vi "Make empty strings null.vi"(11 "JSON Input":string) -> (3 "<JSON>":string)   [LabVIEW 2020, in "JSONtext.lvlib"]
uses:
  <vilib>/JDP Science/JSONtext/JSONtext.lvlib
  <vilib>/JDP Science/JDP Science Common Utilities/JDP Utility.lvlib
panel:
  # "Make empty input count as null"
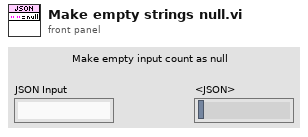
[diagram p1: front panel]
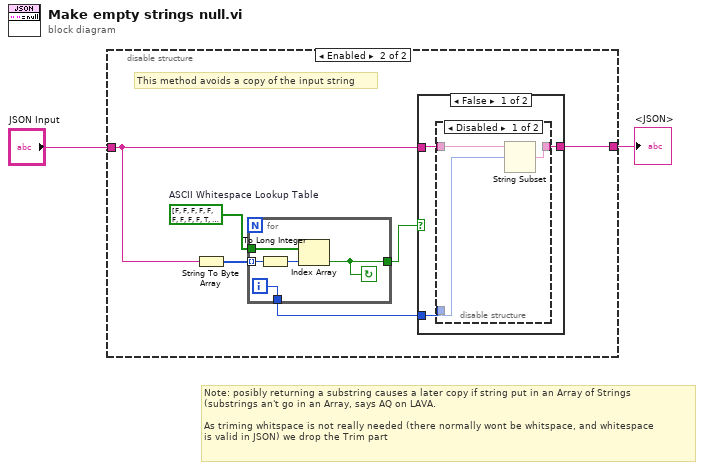
[diagram p0: block diagram]
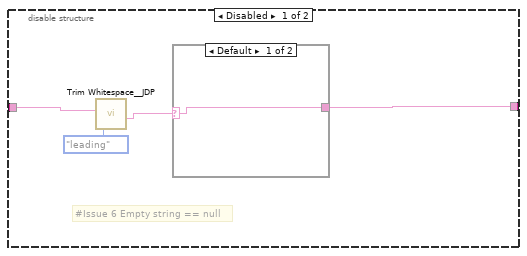
[diagram p2: hidden frame]
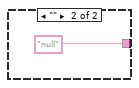
[diagram p3: hidden frame]
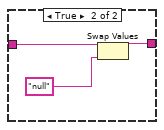
[diagram p5: hidden frame]
diagram:
  # "Note: posibly returning a substring causes a later copy if string put in an Array of Strings\n(substrings an't go in an Array, says AQ on LAVA.\n\nAs triming whitspace is not really needed (there normally wont be whitspace, and whitespace\nis valid in JSON) we drop the Trim part"
  n1 = disable-structure shown="Enabled" {
    disable-tunnel: "JSON Input" -> [w6 w12]
    disable-tunnel: [w4 w11] -> w1
    frame Disabled {
      # "#Issue 6 Empty string == null"
      n2 = call <vilib>:"Trim Whitespace__JDP.vi"("Remove (leading and trailing)"=enum16{"leading", "trailing", "both"}."leading", "String in"=w6) -> ("String out"=w5:string)  [unwired: 5 in]
      n3 = case shown="Default" w5 {
        selector: w5 -> [w7 _]
        tunnel: [w7 "null"] -> w4
        frame Default {
        }
        frame "" {
        }
      }
    }
    frame Enabled {
      w14 = bool[] [FALSE, FALSE, FALSE, FALSE, FALSE, FALSE, FALSE, FALSE, FALSE, TRUE, TRUE, TRUE, TRUE, TRUE, FALSE, FALSE, FALSE, FALSE, FALSE, FALSE, FALSE, FALSE, FALSE, FALSE, FALSE, FALSE, FALSE, FALSE, FALSE, FALSE, FALSE, FALSE, TRUE]  # ASCII Whitespace Lookup Table
      # "This method avoids a copy of the input string"
      n4 = String To Byte Array(string=w12) -> (unsigned byte array=w13:u8[])
      n5 = for {
        tunnel: w13 -> [w28] mode=indexing
        tunnel: w14 -> [w29]
        tunnel: [w26] -> w10
        tunnel: [w25] -> w9
        i -> [w25]
        stop <- w26 continue-if-true
        n6 = To Long Integer(number=w28) -> (32bit integer=w27:i32)
        n7 = Index Array(array=w29, index=w27) -> (element=w26:bool)
      }
      n8 = case shown="False" w10 {
        tunnel: w12 -> [w16 w24]
        tunnel: [w17 w23] -> w11
        tunnel: w9 -> [w15 _]
        frame False {
          n9 = disable-structure shown="Disabled" {
            disable-tunnel: [w20 w21] -> w17
            disable-tunnel: w16 -> [w19 w21]
            disable-tunnel: w15 -> [w18 _]
            frame Disabled {
              n10 = String Subset(string=w19, offset (0)=w18) -> (substring=w20:string)  [unwired: 1 in]
            }
            frame Enabled {
            }
          }
        }
        frame True {
          n11 = Swap Values(12:w24, 14:"null") -> (1:w23:string)  [unwired: 1 in, 1 out]
        }
      }
    }
  }
  "<JSON>" <- w1
